vi "Connect Execution View.vi"(8 "error in (no error)":errorcluster, 10 "View Control":refnum<k7>, 11 "Seq Manager":refnum<k7>) -> (0 "error out":errorcluster)   [LabVIEW 2014, in "teststand-api.lvlib" / "teststand-api.lvclass"]
uses:
  teststand-api.lvclass
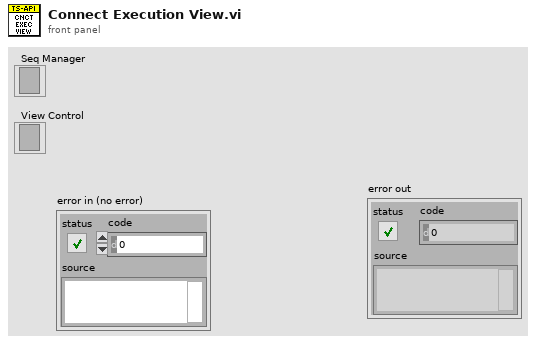
[diagram p1: front panel]
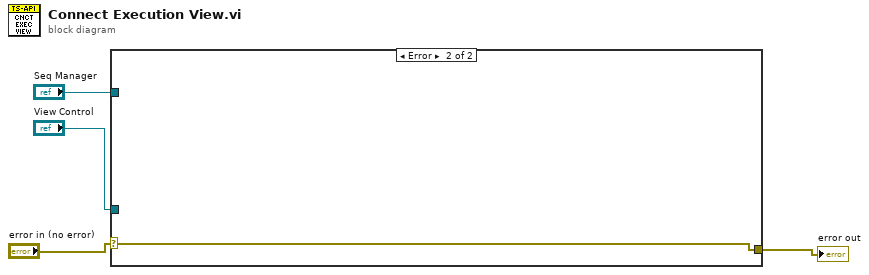
[diagram p0: block diagram]
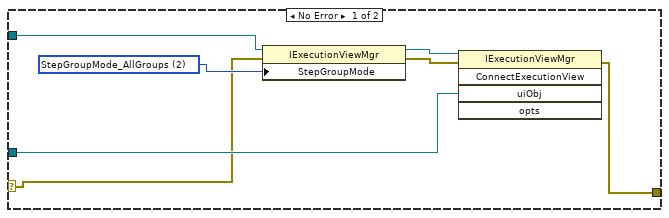
[diagram p2: hidden frame]
diagram:
  n1 = case shown="Error" "error in (no error)" {
    selector: "error in (no error)" -> [w5 w12]
    tunnel: "View Control" -> [w11 _]
    tunnel: "Seq Manager" -> [w8 _]
    tunnel: [w7 w12] -> w1
    frame No Error {
      w6 = 2 items=["StepGroupMode_OneGroup"=1, "StepGroupMode_AllGroups"=2] ("StepGroupMode")
      n2 = property class="IExecutionViewMgr"(reference=w8, error in=w5, "StepGroupMode"=w6) -> (reference out=w9:refnum<k7>, error out=w10:errorcluster)
      n3 = invoke class="IExecutionViewMgr" method="ConnectExecutionView"(reference=w9, error in=w10, "uiObj"=w11) -> (error out=w7:errorcluster)  [unwired: 2 in, 4 out]
    }
    frame Error {
    }
  }
  "error out" <- w1
